vi "from string 1.0.vi"(8 "error in (no error)":errorcluster, 10 "data":string, 11 "ResultProcessor Config in":refnum<class "ResultProcessor Config.lvclass">) -> (0 "error out":errorcluster, 3 "ResultProcessor Config out":refnum<class "ResultProcessor Config.lvclass">)   [LabVIEW 2015, in "ResultProcessor Config.lvclass"]
uses:
  ResultProcessor Config.lvclass
  Report/Generic/Config/Report Config.lvclass
  Report/On-The-Fly/Config/OnTheFlyReport Config.lvclass
  ResultProcessor Config.lvclass/ResultProcessor Config.ctl
  <vilib>/NI/Configuration Framework/serializable configuration/NISE_CEF_serializable configuration.lvclass
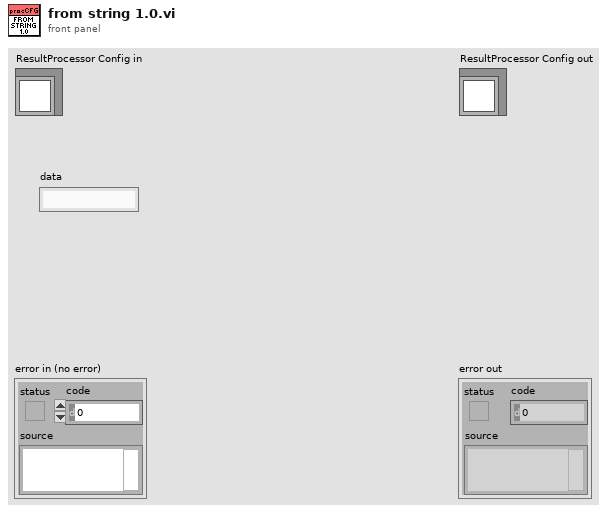
[diagram p1: front panel]
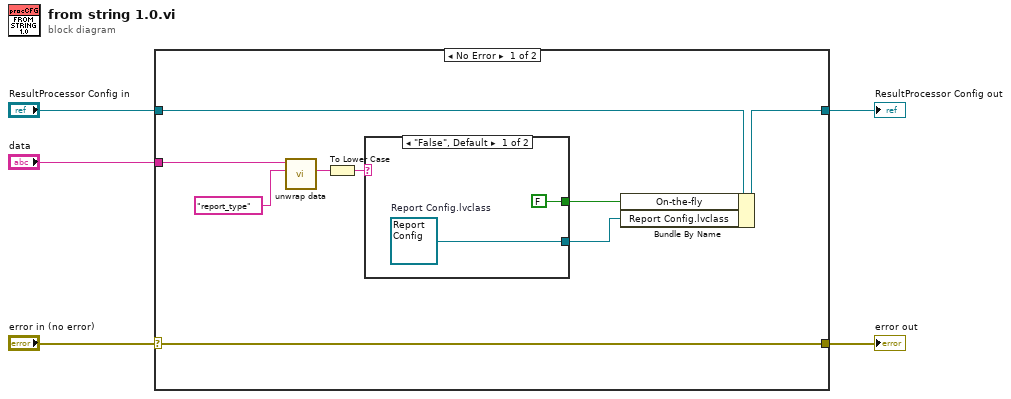
[diagram p0: block diagram]
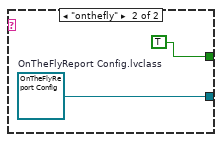
[diagram p2: hidden frame]
diagram:
  n1 = case shown="No Error" "error in (no error)" {
    selector: "error in (no error)" -> [w14 w20]
    tunnel: [w14 w20] -> w4
    tunnel: [w12 w19] -> w2
    tunnel: "ResultProcessor Config in" -> [w13 w19]
    tunnel: "data" -> [w11 _]
    frame No Error {
      n2 = call <vilib>:"unwrap data.vi"("identifier"="report_type", "data to unwrap"=w11) -> ("unwrapped data"=w8:string)  [unwired: 8 in, 1 out]
      n3 = To Lower Case(string=w8) -> (all lower case string=w6:string)
      n4 = case shown="\"False\", Default" w6 {
        tunnel: [w16 w18] -> w10
        tunnel: [FALSE TRUE] -> w9
        frame "False", Default {
          w16 = refnum<class "Report Config.lvclass"> refnum  # Report Config.lvclass
        }
        frame "onthefly" {
          w18 = refnum<class "OnTheFlyReport Config.lvclass"> refnum  # OnTheFlyReport Config.lvclass
        }
      }
      n5 = Bundle By Name(cluster=w13, "On-the-fly"=w9, "Report Config.lvclass"=w10) -> (w12:refnum<class "ResultProcessor Config.lvclass">)
    }
    frame Error {
    }
  }
  "error out" <- w4
  "ResultProcessor Config out" <- w2
